vi "Included.vi"(11 "Type in":refnum<class "Type.lvclass">) -> (2 "Included":bool)   [LabVIEW 2020, in "Conditu2.lvlib" / "Columns.lvlib" / "Type.lvclass"]
uses:
  Type.lvclass
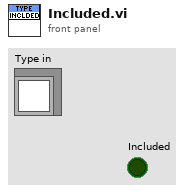
[diagram p1: front panel]
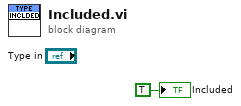
[diagram p0: block diagram]
diagram:
  "Included" <- TRUE ("Included")
